vi "Synchronize-Start.vi"() -> ()   [LabVIEW 2020]
uses:
  <vilib>/Platform/TimedLoop/XDataNode/wakeup.ctl
  <vilib>/Platform/TimedLoop/XDataNode/XDNodeRunTimeDep.lvlib
  <vilib>/Platform/TimedLoop/XDataNode/nitl_modes.ctl
  <vilib>/Platform/TimedLoop/XDataNode/timing_clust.ctl
  <vilib>/Platform/TimedLoop/XDataNode/XDataNode.xnode
panel:
  in  "stop":bool
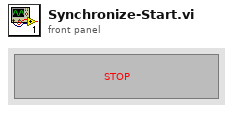
[diagram p1: front panel]
types:
  T1 = typedef "XDNodeRunTimeDep.lvlib/timing_clust.ctl" = cluster{"Expected End [f-1]":u64, "Actual End [f-1]":u64, "Finished Late? [f-1]":bool, "Expected End [i-1]":u64, "Actual End [i-1]":u64, "Finished Late? [i-1]":bool, "Expected Start [i]":u64, "Actual Start [i]":u64, "Expected Start [f]":u64, "Actual Start [f]":u64, "Source Name":string, "Structure Name":string, "Period":i64, "Deadline":i64, "Offset":i64, "Start":i64, "Priority":i32, "Timeout":i32, "Mode":T2, "Wakeup Reason":T3, "Error":errorcluster, "Source Type":string, "Secondary Source Type":string, "Global End Time":u64, "Global Start Time":u64, "Frame Duration":u64, "Iteration Duration":u64, "Assigned CPU":i32, "I/O Scan Engine Mode":u32}
  T2 = typedef "XDNodeRunTimeDep.lvlib/nitl_modes.ctl" = enum32{"No Change", "Process missed periods, maintain original phase", "Discard missed periods, maintain original phase", "Process missed periods, ignore original phase", "Discard missed periods, ignore original phase"}
  T3 = typedef "XDNodeRunTimeDep.lvlib/wakeup.ctl" = enum32{"Normal", "Aborted", "Asynchronous wakeup", "Timing source error", "Timed loop error", "Timeout"}
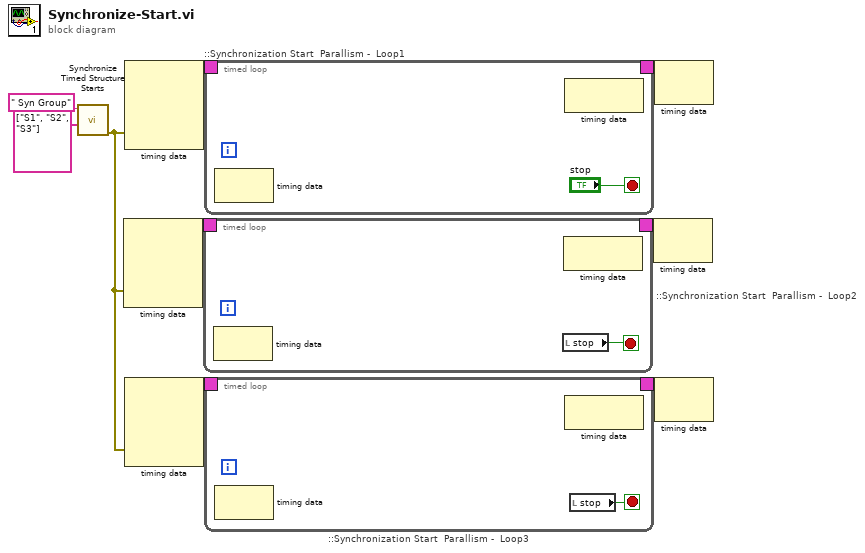
[diagram p0: block diagram]
diagram:
  n1 = call <vilib>:"Synchronize Timed Structure Starts.vi"("timed structure names"=string[] ["S1", "S2", "S3"], "synchronization group name"=" Syn Group") -> ("error out"=w2:errorcluster)  [unwired: 8 in, 1 out]
  n2 = node-c288(w2) -> (w6:T1)  [unwired: 3 in]
  n3 = node-c288(w2) -> (w9:T1)  [unwired: 3 in]
  n4 = node-c288(w2) -> (w4:T1)  [unwired: 3 in]
  n5 = timed-loop "::Synchronization Start  Parallism -  Loop2" {
    timing: w6 -> [_]
    timing-out: [_] -> w5
    stop <- w10 stop-if-true
    n6 = node-c288() -> ()  [unwired: 1 in, 1 out]
    n7 = local read "stop"() -> (w10:bool)
    n8 = node-c288() -> ()  [unwired: 1 in, 1 out]
  }
  n9 = timed-loop "::Synchronization Start  Parallism -  Loop1" {
    timing: w9 -> [_]
    timing-out: [_] -> w8
    stop <- "stop" stop-if-true
    n10 = node-c288() -> ()  [unwired: 1 in, 1 out]
    n11 = node-c288() -> ()  [unwired: 1 in, 1 out]
  }
  n12 = timed-loop "::Synchronization Start  Parallism -  Loop3" {
    timing: w4 -> [_]
    timing-out: [_] -> w3
    stop <- w16 stop-if-true
    n13 = node-c288() -> ()  [unwired: 1 in, 1 out]
    n14 = node-c288() -> ()  [unwired: 1 in, 1 out]
    n15 = local read "stop"() -> (w16:bool)
  }
  n16 = node-c288(w5) -> ()  [unwired: 1 out]
  n17 = node-c288(w8) -> ()  [unwired: 1 out]
  n18 = node-c288(w3) -> ()  [unwired: 1 out]
